vi "niRFUtil MEAS Multiply and Add (real wfms).vi"(0 "Waveform 1 In":T1 {"y" min=0 max=127 format="%.2f"; "dx" format="%^.2e"; "x0" format="%^.2e"}, 5 "Waveform 2 In":T1 {"y" min=0 max=127 format="%.2f"; "dx" format="%^.2e"; "x0" format="%^.2e"}) -> (4 "Multiply and Add":sgl format="%.2g", 6 "x0":dbl format="%.2g", 8 "dx":dbl format="%.2g", 10 "Max value":sgl format="%.2p", 15 "Max index":i32)   [LabVIEW 2015, in "niRFUtil.lvlib"]
uses:
  niRFUtil.lvlib
  Includes/niRFUtil INC Real Waveform.ctl
  Includes/niRFUtil INC Real Array.ctl
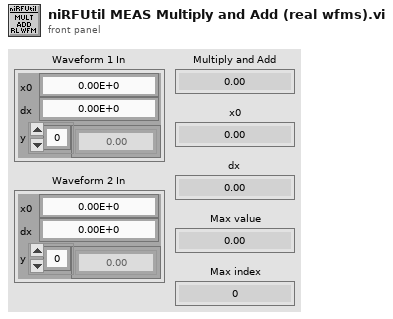
[diagram p1: front panel]
types:
  T1 = typedef "niRFUtil.lvlib/niRFUtil INC Real Waveform.ctl" = cluster{"x0":dbl, "dx":dbl, "y":T2}
  T2 = typedef "niRFUtil.lvlib/niRFUtil INC Real Array.ctl" = sgl[]
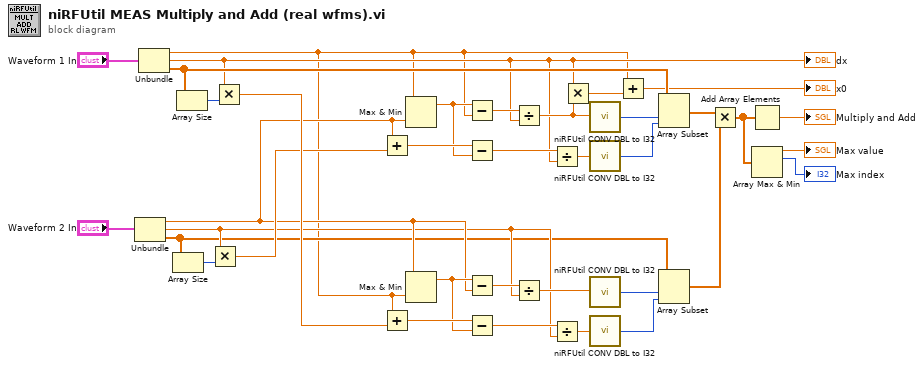
[diagram p0: block diagram]
diagram:
  n1 = Unbundle("Waveform 2 In") -> ("x0"=w12:dbl, "dx"=w11:dbl, "y"=w10:T2)
  n2 = Unbundle("Waveform 1 In") -> ("x0"=w5:dbl, "dx"=w7:dbl, "y"=w13:T2)
  "dx" <- w7
  n3 = Array Size(array=w10) -> (size(s)=w36:i32)
  n4 = Array Size(array=w13) -> (size(s)=w35:i32)
  n5 = Multiply(x=w11, y=w36) -> (x*y=w23:dbl)
  n6 = Multiply(x=w7, y=w35) -> (x*y=w25:dbl)
  n7 = Add(x=w12, y=w23) -> (x+y=w21:dbl)
  n8 = Add(x=w5, y=w25) -> (x+y=w33:dbl)
  n9 = Max & Min(x=w5, y=w12) -> (max(x,y)=w20:dbl)  [unwired: 1 out]
  n10 = Max & Min(x=w12, y=w5) -> (max(x,y)=w32:dbl)  [unwired: 1 out]
  n11 = Subtract(x=w20, y=w5) -> (x-y=w22:dbl)
  n12 = Subtract(x=w21, y=w20) -> (x-y=w19:dbl)
  n13 = Subtract(x=w32, y=w12) -> (x-y=w34:dbl)
  n14 = Subtract(x=w33, y=w32) -> (x-y=w31:dbl)
  n15 = Divide(x=w22, y=w7) -> (x/y=w8:dbl)
  n16 = Divide(x=w34, y=w11) -> (x/y=w28:dbl)
  n17 = Divide(x=w19, y=w7) -> (x/y=w18:dbl)
  n18 = Divide(x=w31, y=w11) -> (x/y=w30:dbl)
  n19 = Multiply(x=w7, y=w8) -> (x*y=w6:dbl)
  n20 = call "niRFUtil CONV DBL to I32.vi"("Numeric (DBL)"=w8) -> ("Numeric (I32)"=w16:i32)  [unwired: 14 in]
  n21 = call "niRFUtil CONV DBL to I32.vi"("Numeric (DBL)"=w18) -> ("Numeric (I32)"=w17:i32)  [unwired: 14 in]
  n22 = call "niRFUtil CONV DBL to I32.vi"("Numeric (DBL)"=w28) -> ("Numeric (I32)"=w27:i32)  [unwired: 14 in]
  n23 = call "niRFUtil CONV DBL to I32.vi"("Numeric (DBL)"=w30) -> ("Numeric (I32)"=w29:i32)  [unwired: 14 in]
  n24 = Add(x=w5, y=w6) -> (x+y=→"x0":dbl)
  n25 = Array Subset(array=w13, index=w16, length=w17) -> (w14:T2)
  n26 = Array Subset(array=w10, index=w27, length=w29) -> (w15:T2)
  n27 = Multiply(x=w14, y=w15) -> (x*y=w3:T2)
  n28 = Add Array Elements(numeric array=w3) -> (sum=→"Multiply and Add":sgl)
  n29 = Array Max & Min(array=w3) -> (max value=→"Max value":sgl, max index (indices)=→"Max index":i32)  [unwired: 2 out]
